vi "Introspection Core.vi"(8 "error in (no error)":errorcluster, 11 "CS++PPG in":refnum<class "CS++PPG.lvclass">) -> (0 "error out":errorcluster, 2 "CS++Messages":refnum<class "Message.lvclass">[](array[class]), 3 "CS++PPG out":refnum<class "CS++PPG.lvclass">)   [LabVIEW 2016, in "CS++PPG.lvlib" / "CS++PPG.lvclass"]
doc: "This vi delivers a list with all messages this actor reacts to. \n\nNote that all inherited classes have to overwrite it."
uses:
  CS++PPG.lvclass
  <vilib>/ActorFramework/Message/Message.lvclass
  CS++PPG Messages/Set Letter Time Msg/Set Letter Time Msg.lvclass
  C:/Program Files (x86)/National Instruments/LabVIEW 2016/vi.lib/ActorFramework/Message/Message.lvclass
  CS++PPG Messages/Start Pattern Msg/Start Pattern Msg.lvclass
  CS++PPG Messages/Stop Pattern Msg/Stop Pattern Msg.lvclass
  CS++PPG Messages/Load Pattern Msg/Load Pattern Msg.lvclass
  CS++PPG Messages/Set Mode Msg/Set Mode Msg.lvclass
  CSPP_Core/Actors/CS++DeviceActor/CS++DeviceActor.lvclass
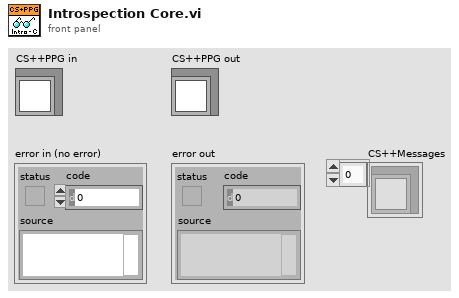
[diagram p1: front panel]
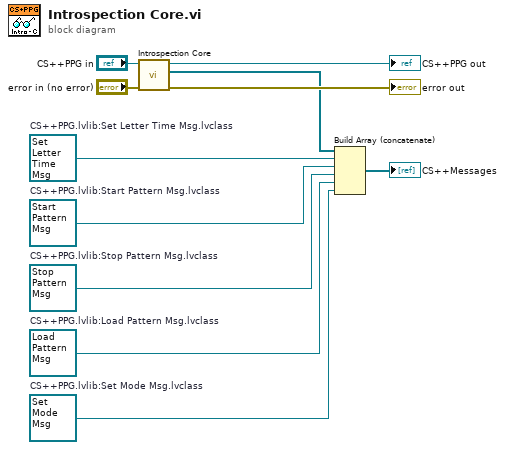
[diagram p0: block diagram]
diagram:
  w1 = refnum<class "Set Mode Msg.lvclass"> refnum  # CS++PPG.lvlib:Set Mode Msg.lvclass
  w2 = refnum<class "Load Pattern Msg.lvclass"> refnum  # CS++PPG.lvlib:Load Pattern Msg.lvclass
  w3 = refnum<class "Stop Pattern Msg.lvclass"> refnum  # CS++PPG.lvlib:Stop Pattern Msg.lvclass
  w4 = refnum<class "Start Pattern Msg.lvclass"> refnum  # CS++PPG.lvlib:Start Pattern Msg.lvclass
  w5 = refnum<class "Set Letter Time Msg.lvclass"> refnum  # CS++PPG.lvlib:Set Letter Time Msg.lvclass
  n1 = call-parent "Introspection Core.vi"("error in (no error)"="error in (no error)", "CS++DeviceActor in"="CS++PPG in") -> ("error out"=→"error out":errorcluster, "CS++Messages"=w7:refnum<class "Message.lvclass">[], "CS++DeviceActor out"=→"CS++PPG out":refnum<class "CS++PPG.lvclass">)  [unwired: 7 in]
  n2 = Build Array (concatenate)(w7, w5, w4, w3, w2, w1) -> (→"CS++Messages":refnum<class "Message.lvclass">[])
